vi "Write Assert.vi"(8 "error in (no error)":errorcluster, 10 "Assert":refnum<class "Assert.lvclass">, 11 "Assert Factory in":refnum<class "Assert Factory.lvclass">) -> (0 "error out":errorcluster, 3 "Assert Factory out":refnum<class "Assert Factory.lvclass">)   [LabVIEW 2009]
uses:
  Assert Factory.lvclass
  Assert/Assert.lvclass
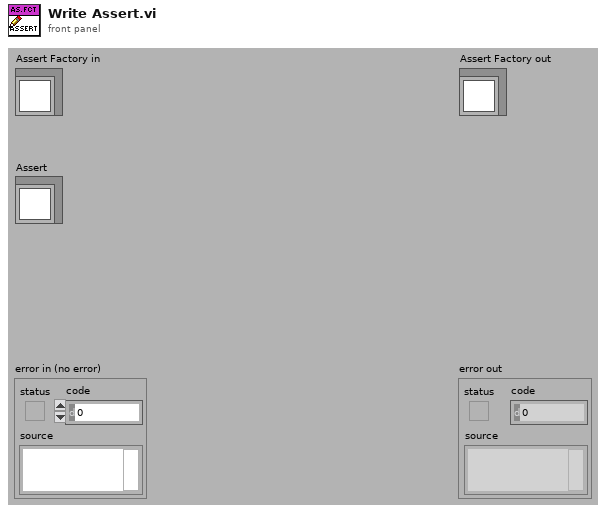
[diagram p1: front panel]
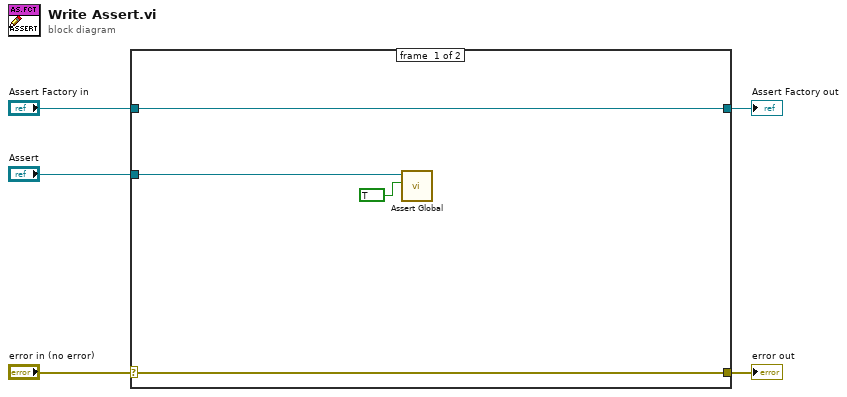
[diagram p0: block diagram]
diagram:
  n1 = case shown="No Error" "error in (no error)" {
    selector: "error in (no error)" -> [w8 w11]
    tunnel: [w8 w11] -> w4
    tunnel: [w9 w10] -> w2
    tunnel: "Assert Factory in" -> [w9 w10]
    tunnel: "Assert" -> [w7 _]
    frame #0 {
      n2 = call "Assert Global.vi"("Set (F)"=TRUE, "Assert in"=w7) -> ()  [unwired: 7 in, 3 out]
    }
    frame #1 {
    }
  }
  "error out" <- w4
  "Assert Factory out" <- w2
